vi "Initialize.vi"(8 "error in":errorcluster, 10 "XYGraph in":refnum<vi>, 11 "GUI In":refnum<class "Calibration UI.lvclass">) -> (0 "error out":errorcluster, 3 "GUI Out":refnum<class "Calibration UI.lvclass">)   [LabVIEW 2015, in "Calibration UI.lvclass"]
uses:
  Calibration UI.lvclass
  Calibration/State data/State Data.lvclass
  Calibration UI.lvclass/Calibration UI.ctl
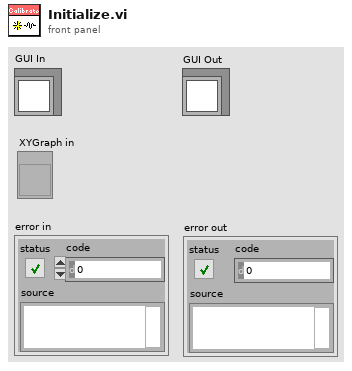
[diagram p1: front panel]
types:
  T1 = cluster{"Stored State":refnum<class "State Data.lvclass">[], "pointer to data":i32}
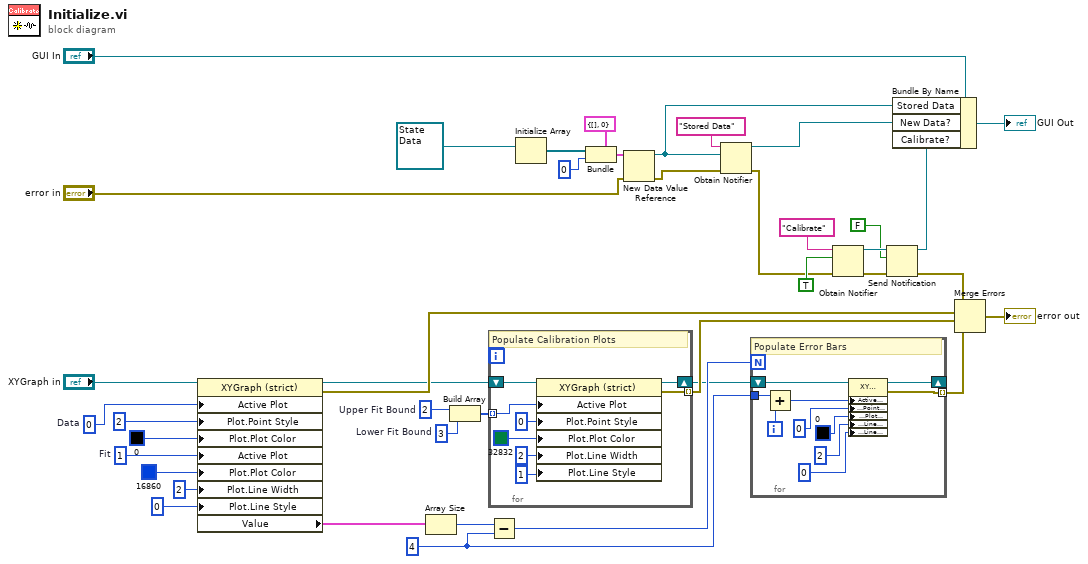
[diagram p0: block diagram]
diagram:
  w35 = 4 ("y")
  w24 = u32 3  # Lower Fit Bound
  w23 = u32 2  # Upper Fit Bound
  w29 = u32 1  # Fit
  w32 = u32 0  # Data
  n1 = property on="Property Node" class="XYGraph (strict)"(reference="XYGraph in", "Active Plot"=w32, "Plot.Point Style"=u8 2, "Plot.Plot Color"=u32 0, "Active Plot"=w29, "Plot.Plot Color"=u32 16860, "Plot.Line Width"=u8 2, "Plot.Line Style"=u8 0) -> (reference out=w25:refnum<vi>, error out=w41:errorcluster, "Value"=w33:cluster{dbl[], "Upper Bound":dbl[]}[])  [unwired: 1 in]
  n2 = Array Size(array=w33) -> (size(s)=w34:i32)
  n3 = Build Array(w23, w24) -> (w22:u32[])
  n4 = for {
    shift-right: [w43] -> w21
    shift-left: w25 -> [w44]
    tunnel: w22 -> [w49] mode=indexing
    tunnel: [w42] -> w38 mode=indexing
    # "Populate Calibration Plots"
    n5 = property on="Property Node" class="XYGraph (strict)"(reference=w44, "Active Plot"=w49, "Plot.Point Style"=u8 0, "Plot.Plot Color"=u32 32832, "Plot.Line Width"=u8 2, "Plot.Line Style"=u8 1) -> (reference out=w43:refnum<vi>, error out=w42:errorcluster)  [unwired: 1 in]
  }
  n6 = Subtract(x=w34, y=w35) -> (x-y=w36:i32)
  n7 = Initialize Array(refnum<class "State Data.lvclass"> refnum ("State Data")) -> (w18:refnum<class "State Data.lvclass">[])  [unwired: 1 in]
  n8 = Bundle(cluster=T1 {"Stored State"=[], "pointer to data"=0} ("Data and Pointer"), "Stored State"=w18, "pointer to data"=0) -> (w19:T1)
  n9 = New Data Value Reference(data value=w19, error in="error in") -> (data value reference=w14:refnum<data-value>, error out=w4:errorcluster)
  n10 = Obtain Notifier(name (unnamed)="Stored Data", notification data type=w14, error in (no error)=w4) -> (notifier out=w12:refnum<notifier>, error out=w3:errorcluster)  [unwired: 1 in, 1 out]
  n11 = for {
    N: w36 -> [_]
    shift-right: [w54] -> _
    shift-left: w21 -> [w55]
    tunnel: w35 -> [w52]
    tunnel: [w50] -> w37 mode=indexing
    i -> [w53]
    # "Populate Error Bars"
    n12 = Add(x=w52, y=w53) -> (x+y=w51:i32)
    n13 = property on="Property Node" class="XYGraph (strict)"(reference=w55, "Active Plot"=w51, "Plot.Point Style"=u8 0, "Plot.Plot Color"=u32 0, "Plot.Line Width"=u8 2, "Plot.Line Style"=u8 0) -> (reference out=w54:refnum<vi>, error out=w50:errorcluster)  [unwired: 1 in]
  }
  n14 = Obtain Notifier(name (unnamed)="Calibrate", notification data type=TRUE, error in (no error)=w3) -> (notifier out=w9:refnum<notifier>, error out=w7:errorcluster)  [unwired: 1 in, 1 out]
  n15 = Send Notification(notification=FALSE, notifier=w9, error in (no error)=w7) -> (notifier out=w6:refnum<notifier>, error out=w1:errorcluster)
  n16 = Bundle By Name(cluster="GUI In", "Stored Data"=w14, "New Data?"=w12, "Calibrate?"=w6) -> (→"GUI Out":refnum<class "Calibration UI.lvclass">)
  n17 = Merge Errors(w1, w41, w38, w37) -> (→"error out":errorcluster)
